vi "Manual Mode Read Vacuum.vi"(8 "error in":errorcluster, 11 "Gantry in":refnum<class "Gantry Class.lvclass">) -> (0 "error out":errorcluster, 2 "Vacuum Status":T1, 3 "Gantry out":refnum<class "Gantry Class.lvclass">)   [LabVIEW 2017]
uses:
  Shared Components/Gantry Class/Gantry Class.lvclass
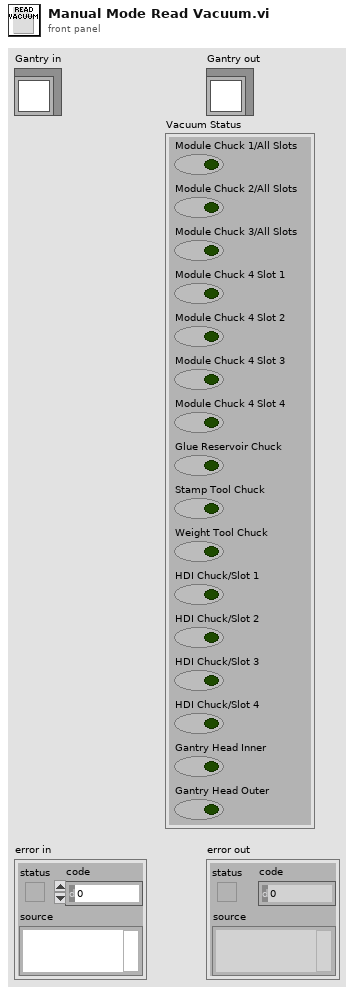
[diagram p1: front panel]
types:
  T1 = cluster{"Module Chuck 1/All Slots":bool, "Module Chuck 2/All Slots":bool, "Module Chuck 3/All Slots":bool, "Module Chuck 4 Slot 1":bool, "Module Chuck 4 Slot 2":bool, "Module Chuck 4 Slot 3":bool, "Module Chuck 4 Slot 4":bool, "Glue Reservoir Chuck":bool, "Stamp Tool Chuck":bool, "Weight Tool Chuck":bool, "HDI Chuck/Slot 1":bool, "HDI Chuck/Slot 2":bool, "HDI Chuck/Slot 3":bool, "HDI Chuck/Slot 4":bool, "Gantry Head Inner":bool, "Gantry Head Outer":bool}
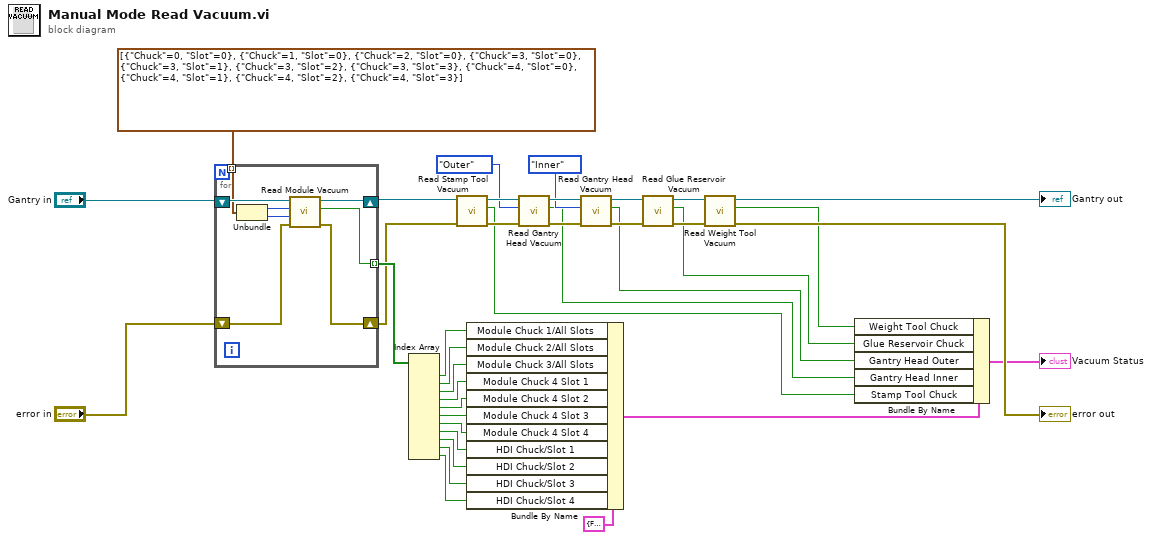
[diagram p0: block diagram]
diagram:
  n1 = for {
    shift-right: [w45] -> w13
    shift-left: "error in" -> [w44]
    tunnel: cluster{"Chuck":i32, "Slot":i32}[] [{"Chuck"=0, "Slot"=0}, {"Chuck"=1, "Slot"=0}, {"Chuck"=2, "Slot"=0}, {"Chuck"=3, "Slot"=0}, {"Chuck"=3, "Slot"=1}, {"Chuck"=3, "Slot"=2}, {"Chuck"=3, "Slot"=3}, {"Chuck"=4, "Slot"=0}, {"Chuck"=4, "Slot"=1}, {"Chuck"=4, "Slot"=2}, {"Chuck"=4, "Slot"=3}] -> [w42] mode=indexing
    shift-right: [w39] -> w18
    shift-left: "Gantry in" -> [w43]
    tunnel: [w38] -> w30 mode=indexing
    n2 = Unbundle(w42) -> ("Chuck"=w41:i32, "Slot"=w40:i32)
    n3 = call-dynamic "Read Module Vacuum.vi"("error in"=w44, "Slot Number"=w40, "Chuck Number"=w41, "Gantry in"=w43) -> ("error out"=w45:errorcluster, "On/Off"=w38:bool, "Gantry out"=w39:refnum<class "Gantry Class.lvclass">)  [unwired: 5 in]
  }
  n4 = Index Array(array=w30) -> (element #1=w29:bool, element #2=w28:bool, element #3=w27:bool, element #4=w26:bool, element #5=w25:bool, element #6=w24:bool, element #7=w23:bool, element #8=w22:bool, element #9=w21:bool, element #10=w20:bool, element #11=w19:bool)  [unwired: 11 in]
  n5 = call-dynamic "Read Stamp Tool Vacuum.vi"("error in"=w13, "Gantry in"=w18) -> ("error out"=w12:errorcluster, "On/Off"=w5:bool, "Gantry out"=w17:refnum<class "Gantry Class.lvclass">)  [unwired: 7 in]
  n6 = Bundle By Name(cluster=T1 {"Module Chuck 1/All Slots"=FALSE, "Module Chuck 2/All Slots"=FALSE, "Module Chuck 3/All Slots"=FALSE, "Module Chuck 4 Slot 1"=FALSE, "Module Chuck 4 Slot 2"=FALSE, "Module Chuck 4 Slot 3"=FALSE, "Module Chuck 4 Slot 4"=FALSE, "Glue Reservoir Chuck"=FALSE, "Stamp Tool Chuck"=FALSE, "Weight Tool Chuck"=FALSE, "HDI Chuck/Slot 1"=FALSE, "HDI Chuck/Slot 2"=FALSE, "HDI Chuck/Slot 3"=FALSE, "HDI Chuck/Slot 4"=FALSE, "Gantry Head Inner"=FALSE, "Gantry Head Outer"=FALSE} ("Vacuum Status"), "Module Chuck 1/All Slots"=w29, "Module Chuck 2/All Slots"=w28, "Module Chuck 3/All Slots"=w27, "Module Chuck 4 Slot 1"=w26, "Module Chuck 4 Slot 2"=w25, "Module Chuck 4 Slot 3"=w24, "Module Chuck 4 Slot 4"=w23, "HDI Chuck/Slot 1"=w22, "HDI Chuck/Slot 2"=w21, "HDI Chuck/Slot 3"=w20, "HDI Chuck/Slot 4"=w19) -> (w6:T1)
  n7 = call-dynamic "Read Gantry Head Vacuum.vi"("error in"=w12, "Inner/Outer"=enum16{"Outer", "Inner"}."Outer", "Gantry in"=w17) -> ("error out"=w11:errorcluster, "On/Off"=w4:bool, "Gantry out"=w16:refnum<class "Gantry Class.lvclass">)  [unwired: 6 in]
  n8 = call-dynamic "Read Gantry Head Vacuum.vi"("error in"=w11, "Inner/Outer"=enum16{"Outer", "Inner"}."Inner", "Gantry in"=w16) -> ("error out"=w10:errorcluster, "On/Off"=w3:bool, "Gantry out"=w15:refnum<class "Gantry Class.lvclass">)  [unwired: 6 in]
  n9 = call-dynamic "Read Glue Reservoir Vacuum.vi"("error in"=w10, "Gantry in"=w15) -> ("error out"=w9:errorcluster, "On/Off"=w2:bool, "Gantry out"=w14:refnum<class "Gantry Class.lvclass">)  [unwired: 7 in]
  n10 = call-dynamic "Read Weight Tool Vacuum.vi"("error in"=w9, "Gantry in"=w14) -> ("error out"=→"error out":errorcluster, "On/Off"=w1:bool, "Gantry out"=→"Gantry out":refnum<class "Gantry Class.lvclass">)  [unwired: 7 in]
  n11 = Bundle By Name(cluster=w6, "Weight Tool Chuck"=w1, "Glue Reservoir Chuck"=w2, "Gantry Head Outer"=w3, "Gantry Head Inner"=w4, "Stamp Tool Chuck"=w5) -> (→"Vacuum Status":T1)
